vi "Window_Size.vi"() -> ()   [LabVIEW 2020]
panel:
  out "Window_Size":i64
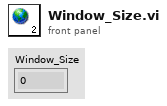
[diagram p1: front panel]
diagram:
